vi "GetProcessReference.vi"(8 "error in (no error)":errorcluster, 11 "EmbeddedSMO in":refnum<class "SMO.UI.Embedded.lvclass">) -> (0 "error out":errorcluster, 2 "Static VI Ref":refnum<vi>, 3 "EmbeddedSMO out":refnum<class "SMO.UI.Embedded.lvclass">)   [LabVIEW 2016, in "SMO.UI.Embedded.lvclass"]
uses:
  SMO.UI.Embedded.lvclass
  C:/Program Files (x86)/National Instruments/LabVIEW 2016/vi.lib/JKI/JKI SMO/SMO/SMO.lvclass
  <vilib>/JKI/JKI SMO/SMO/SMO.lvclass
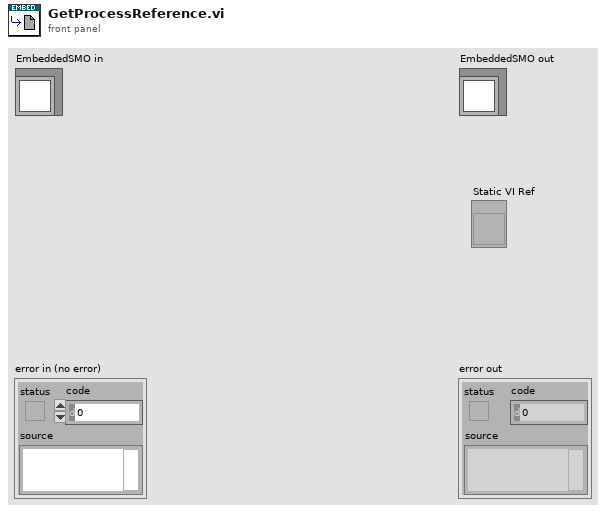
[diagram p1: front panel]
types:
  T1 = typedef "SMO.lvclass/RegisteredProcessData--Cluster.ctl" = cluster{"Name":string, "Static VI Ref":refnum<vi>, "Running":bool, "NotifierRef":u32}
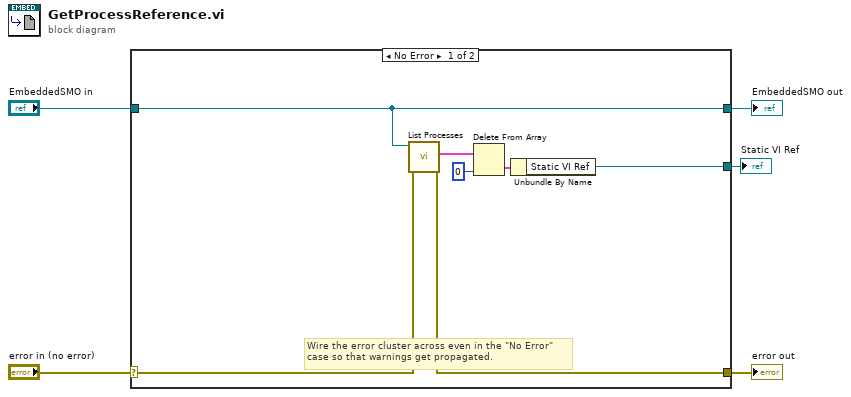
[diagram p0: block diagram]
diagram:
  n1 = case shown="No Error" "error in (no error)" {
    selector: "error in (no error)" -> [w7 w14]
    tunnel: [w6 w14] -> w4
    tunnel: [w12 w13] -> w2
    tunnel: "EmbeddedSMO in" -> [w12 w13]
    tunnel: [w8 _] -> w1
    frame No Error {
      # "Wire the error cluster across even in the \"No Error\"\ncase so that warnings get propagated."
      n2 = call <vilib>:"List Processes.vi"("error in (no error)"=w7, "SMO"=w12) -> ("error out"=w6:errorcluster, "Registered Processes"=w11:T1[])  [unwired: 7 in, 1 out]
      n3 = Delete From Array(array=w11, index=0) -> (deleted portion=w9:T1)  [unwired: 1 in, 1 out]
      n4 = Unbundle By Name(w9) -> ("Static VI Ref"=w8:refnum<vi>)
    }
    frame Error {
    }
  }
  "error out" <- w4
  "EmbeddedSMO out" <- w2
  "Static VI Ref" <- w1
